vi "Send Configure Relays.vi"(5 "Alarm Type (0:Low)":u16(ring) items=["Low", "High", "Both"], 6 "Mode (0:Off)":enum16{"Off", "On", "Alarms"}(ring), 7 "Message Priority (Normal)":T1=enum."Normal", 8 "error in (no error)":errorcluster, 9 "Input (0)":i32 min=0 max=7 step=1, 10 "Relay (0)":i32=1 min=0 max=7 step=1, 11 "Message Enqueuer":refnum<class "Message Enqueuer.lvclass">) -> (0 "error out":errorcluster, 3 "Message Enqueuer out":refnum<class "Message Enqueuer.lvclass">)   [LabVIEW 2016, in "LS218.lvlib" / "Configure Relays Msg.lvclass"]
doc: "Sends the <B>LS218.lvlib:Configure Relays Msg.lvclass</B> message.\n\n<B>LS218.lvlib:LS218.lvclass:Configure Relays.vi</B> Description:\n\nThis VI configures relay paramters. Relays may be configured manually or set to activate on an input alarm condition. Only the model 218S includes the relays."
uses:
  Configure Relays Msg.lvclass
  <vilib>/ActorFramework/Message Enqueuer/Message Enqueuer.lvclass
  <vilib>/ActorFramework/Message Enqueuer/Message Priority.ctl
  C:/Program Files (x86)/National Instruments/LabVIEW 2016/vi.lib/ActorFramework/Message/Message.lvclass
  Configure Relays Msg.lvclass/Configure Relays Msg.ctl
  <vilib>/ActorFramework/Message Enqueuer/Message Enqueuer.lvclass/Message Enqueuer.ctl
  <vilib>/ActorFramework/Message Priority Queue/Priority Enqueue.vi
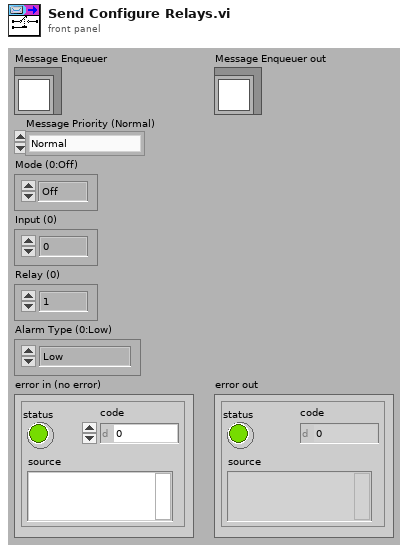
[diagram p1: front panel]
types:
  T1 = typedef "Actor Framework.lvlib/Message Enqueuer.lvclass/Message Priority.ctl" = enum16{"Low", "Normal", "High"}
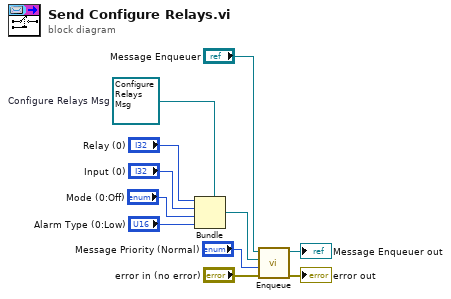
[diagram p0: block diagram]
diagram:
  w5 = refnum<class "Configure Relays Msg.lvclass"> refnum  # Configure Relays Msg
  n1 = Bundle(cluster=w5, "Relay (0)", "Input (0)", "Mode (0:Off)", "Alarm Type (0:Low)") -> (w8:refnum<class "Configure Relays Msg.lvclass">)
  n2 = call <vilib>:"Enqueue.vi"("error in (no error)"="error in (no error)", "Message Priority (Normal)"="Message Priority (Normal)", "Message"=w8, "Message Enqueuer in"="Message Enqueuer") -> ("error out"=→"error out":errorcluster, "Message Enqueuer out"=→"Message Enqueuer out":refnum<class "Message Enqueuer.lvclass">)  [unwired: 6 in]
